vi "send_burleighPairedPulse-v02.vi"(0 "daq_ao":tag="Dev1/ao1", 1 "daq_ai":tag="Dev1/ai0:1", 2 "Jump Polarity":bool, 5 "PairedPulseValuesCluster":T2, 7 "Sample Freq (Hz)":dbl min=0.0 max=40000.0, 12 "Jump Filter Freq (Hz)":dbl=20.0 min=0.0 max=40000.0, 13 "Number of Replicates":i16=1 min=1 max=10, 14 "error in":errorcluster) -> (4 "output cluster":T1, 6 "output waveform":waveform(dbl)[](graph), 8 "protocol response":waveform(dbl)[](graph) caption="jumptestMonitor", 10 "error out":errorcluster)   [LabVIEW 2019]
uses:
  <vilib>/Analysis/3filter.llb/Filter Passband Type.ctl
  <vilib>/Analysis/3filter.llb/Bessel Filter (DBL).vi
  <vilib>/measure/NI_MABase.lvlib
  <vilib>/Analysis/NI_AALBase.lvlib
panel:
  # "doesnt do replicating sweeps, just one go..."
  # "Low"
  # "High"
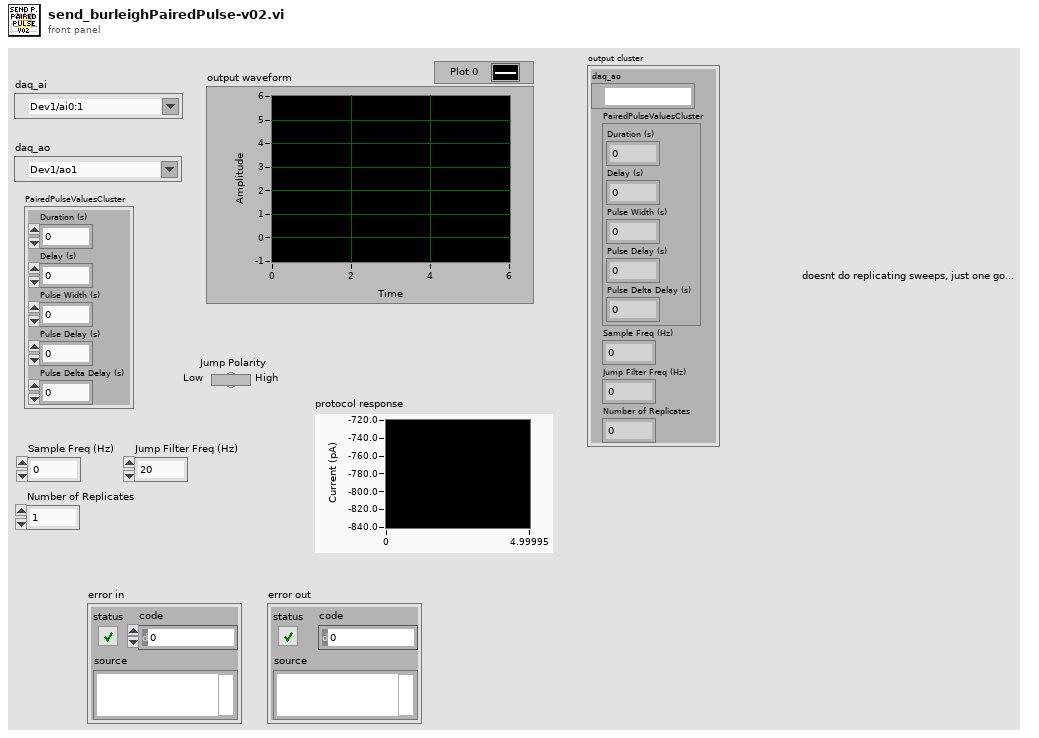
[diagram p1: front panel]
types:
  T1 = cluster{"daq_ao":tag, "PairedPulseValuesCluster":cluster{"Duration (s)":dbl, "Delay (s)":dbl, "Pulse Width (s)":dbl, "Pulse Delay (s)":dbl, "Pulse Delta Delay (s)":dbl}, "Sample Freq (Hz)":dbl, "Jump Filter Freq (Hz)":dbl, "Number of Replicates":i16}
  T2 = cluster{"Duration (s)":dbl, "Delay (s)":dbl, "Pulse Width (s)":dbl, "Pulse Delay (s)":dbl, "Pulse Delta Delay (s)":dbl}
  T3 = typedef "NI_AALBase.lvlib/Filter Passband Type.ctl" = enum32{"Lowpass", "Highpass", "Bandpass", "Bandstop"}
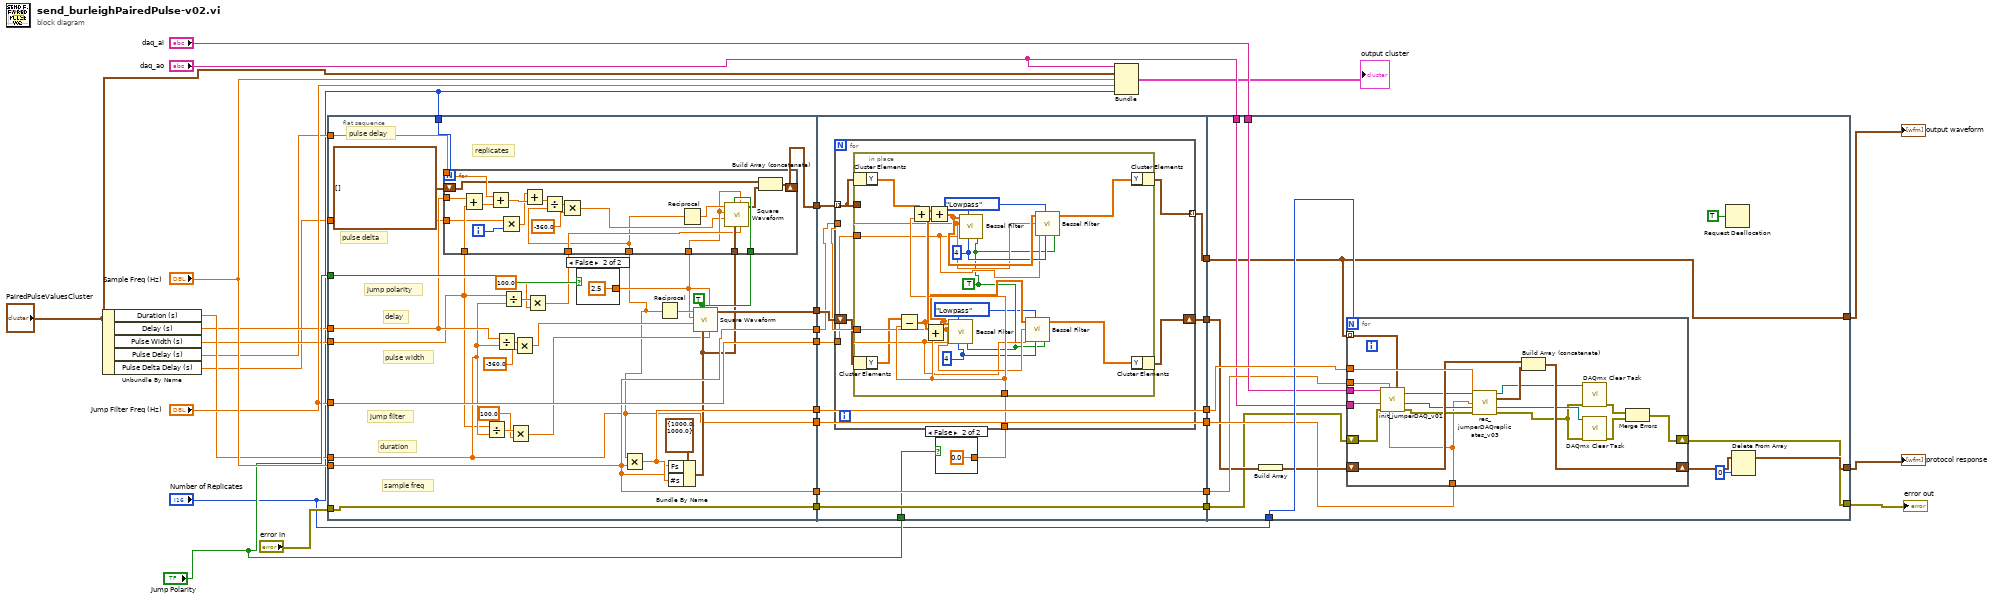
[diagram p0: block diagram]
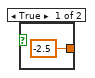
[diagram p2: hidden frame]
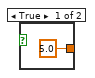
[diagram p3: hidden frame]
diagram:
  n1 = Unbundle By Name("PairedPulseValuesCluster") -> ("Duration (s)"=w10:dbl, "Delay (s)"=w9:dbl, "Pulse Width (s)"=w8:dbl, "Pulse Delay (s)"=w4:dbl, "Pulse Delta Delay (s)"=w2:dbl)
  n2 = flat-sequence {
    tunnel: w10 -> [w34]
    tunnel: "Jump Filter Freq (Hz)" -> [w57]
    tunnel: "Sample Freq (Hz)" -> [w56]
    tunnel: [w58] -> w26
    tunnel: [w56] -> w23
    tunnel: [w57] -> w21
    tunnel: [w56] -> w20
    tunnel: [w55] -> w19
    tunnel: "error in" -> [w54]
    tunnel: [w54] -> w16
    tunnel: "Jump Polarity" -> [w53]
    tunnel: [w34] -> w12
    tunnel: w9 -> [w38]
    tunnel: w8 -> [w33]
    tunnel: [w43] -> w7
    tunnel: w4 -> [w37]
    tunnel: "Number of Replicates" -> [w36]
    tunnel: w2 -> [w35]
    tunnel: w26 -> [w94]
    tunnel: [w94] -> w25
    tunnel: [w92] -> w24
    tunnel: w23 -> [w93]
    tunnel: [w93] -> w22
    tunnel: w21 -> [w86]
    tunnel: w20 -> [w87]
    tunnel: w19 -> [w91]
    tunnel: [w90] -> w17
    tunnel: w16 -> [w90]
    tunnel: "Jump Polarity" -> [w89]
    tunnel: w12 -> [w88]
    tunnel: [w88] -> w11
    tunnel: w7 -> [w84]
    tunnel: [w83] -> w1
    tunnel: [w123] -> w31
    tunnel: w25 -> [w134]
    tunnel: w24 -> [w125]
    tunnel: "daq_ai" -> [w127]
    tunnel: "daq_ao" -> [w124]
    tunnel: w22 -> [w126]
    tunnel: [w130] -> w28
    tunnel: "Number of Replicates" -> [w133]
    tunnel: [w122] -> w15
    tunnel: w17 -> [w121]
    tunnel: w11 -> [w128]
    tunnel: w1 -> [w123]
    frame #0 {
      w47 = TRUE ("reset signal")
      # "replicates"
      # "sample freq"
      # "duration"
      # "jump filter"
      # "pulse width"
      # "delay"
      # "jump polarity"
      # "pulse delta"
      # "pulse delay"
      n3 = Divide(x=w33, y=w34) -> (x/y=w52:dbl)
      n4 = Divide(x=w38, y=w34) -> (x/y=w49:dbl)
      n5 = Divide(x=w33, y=w34) -> (x/y=w45:dbl)
      n6 = Multiply(x=w52, y=100.0) -> (x*y=w41:dbl)
      n7 = Multiply(x=w49, y=-360.0) -> (x*y=w46:dbl)
      n8 = Multiply(x=w45, y=100.0) -> (x*y=w40:dbl)
      n9 = case shown="False" w53 {
        tunnel: [-2.5 ("Amplitude") 2.5 ("Amplitude")] -> w39
        frame True {
        }
        frame False {
        }
      }
      n10 = Multiply(x=w34, y=w56) -> (x*y=w58:dbl)
      n11 = Reciprocal(x=w34) -> (1/x=w48:dbl)
      n12 = Bundle By Name(cluster=cluster{"Fs":dbl, "#s":dbl} {"Fs"=1000.0, "#s"=1000.0} ("sampling info"), "Fs"=w56, "#s"=w58) -> (w42:cluster{"Fs":dbl, "#s":dbl})
      n13 = for {
        N: w36 -> [_]
        tunnel: w47 -> [w80]
        tunnel: w42 -> [w79]
        tunnel: w40 -> [w77]
        tunnel: w39 -> [w76]
        tunnel: w33 -> [w71]
        tunnel: w38 -> [w70]
        tunnel: w37 -> [w69]
        tunnel: w34 -> [w67]
        shift-right: [w65] -> w43
        shift-left: waveform(dbl)[] [] -> [w64]
        tunnel: w35 -> [w60]
        i -> [w62]
        n14 = Add(x=w70, y=w71) -> (x+y=w74:dbl)
        n15 = Add(x=w69, y=w74) -> (x+y=w75:dbl)
        n16 = Multiply(x=w60, y=w62) -> (x*y=w61:dbl)
        n17 = Add(x=w61, y=w75) -> (x+y=w63:dbl)
        n18 = Divide(x=w63, y=w67) -> (x/y=w73:dbl)
        n19 = Multiply(x=w73, y=-360.0) -> (x*y=w72:dbl)
        n20 = Reciprocal(x=w67) -> (1/x=w78:dbl)
        n21 = call <vilib>:"Square Waveform.vi"("duty cycle (%)"=w77, "offset"=w76, "sampling info"=w79, "reset signal"=w80, "phase"=w72, "amplitude"=w76, "frequency"=w78) -> ("signal out"=w66:waveform(dbl))  [unwired: 3 in, 1 out]
        n22 = Build Array (concatenate)(w64, w66) -> (w65:waveform(dbl)[])
      }
      n23 = call <vilib>:"Square Waveform.vi"("duty cycle (%)"=w41, "offset"=w39, "sampling info"=w42, "reset signal"=w47, "phase"=w46, "amplitude"=w39, "frequency"=w48) -> ("signal out"=w55:waveform(dbl))  [unwired: 3 in, 1 out]
    }
    frame #1 {
      n24 = case shown="False" w89 {
        tunnel: [5.0 ("Amplitude") 0.0 ("Amplitude")] -> w85
        frame True {
        }
        frame False {
        }
      }
      n25 = for {
        tunnel: w87 -> [w100]
        tunnel: w86 -> [w99]
        tunnel: w85 -> [w101]
        tunnel: w84 -> [w98] mode=indexing
        shift-right: [w95] -> w92
        shift-left: w91 -> [w96]
        tunnel: [w97] -> w83 mode=indexing
        n26 = in-place {
          in-place-border: w98 -> [_]
          in-place-border: w101 -> [w115]
          in-place-border: w100 -> [w110]
          in-place-border: w99 -> [w109]
          w107 = TRUE ("init/cont (init:F)")
          w112 = 4 ("order")
          w113 = Filter_Passband_Type."Lowpass" ("filter type")
          w108 = 4 ("order")
          w106 = Filter_Passband_Type."Lowpass" ("filter type")
          n27 = in-place-cluster #1(w98) -> ("Y"=w105:dbl[])
          n28 = in-place-cluster #2(w96) -> ("Y"=w103:dbl[])
          n29 = Subtract(x=w103, y=w115) -> (x-y=w116:dbl[])
          n30 = Add(x=w105, y=w115) -> (x+y=w117:dbl[])
          n31 = Add(x=w116, y=w115) -> (x+y=w111:dbl[])
          n32 = Add(x=w117, y=w116) -> (x+y=w114:dbl[])
          n33 = call-poly <vilib>:"Bessel Filter.vi"("init/cont (init:F)"=w107, "order"=w108, "filter type"=w106, "low cutoff freq: fl"=w109, "sampling freq: fs"=w110, "X"=w111) -> ()  [unwired: 2 in, 2 out]
          n34 = call-poly <vilib>:"Bessel Filter.vi"("init/cont (init:F)"=w107, "order"=w112, "filter type"=w113, "low cutoff freq: fl"=w109, "sampling freq: fs"=w110, "X"=w114) -> ()  [unwired: 2 in, 2 out]
          n35 = call-poly <vilib>:"Bessel Filter.vi"("init/cont (init:F)"=w107, "order"=w108, "filter type"=w106, "low cutoff freq: fl"=w109, "sampling freq: fs"=w110, "X"=w111) -> ("Filtered X"=w102:dbl[])  [unwired: 2 in, 1 out]
          n36 = call-poly <vilib>:"Bessel Filter.vi"("init/cont (init:F)"=w107, "order"=w112, "filter type"=w113, "low cutoff freq: fl"=w109, "sampling freq: fs"=w110, "X"=w114) -> ("Filtered X"=w104:dbl[])  [unwired: 2 in, 1 out]
          n37 = in-place-cluster #1("Y"=w104) -> (w97:waveform(dbl))
          n38 = in-place-cluster #2("Y"=w102) -> (w95:waveform(dbl))
        }
      }
    }
    frame #2 {
      n39 = Build Array(w125) -> (w132:waveform(dbl)[])
      n40 = for {
        N: w133 -> [_]
        tunnel: w134 -> [w153]
        shift-right: [w151] -> w131
        shift-left: w132 -> [w150]
        tunnel: w128 -> [w143]
        tunnel: w127 -> [w149]
        tunnel: w126 -> [w148]
        tunnel: w124 -> [w147]
        tunnel: w123 -> [w142] mode=indexing
        shift-right: [w139] -> w122
        shift-left: w121 -> [w138]
        n41 = call "init_jumperDAQ_v01.vi"("protocol waveform"=w142, "Duration (s)"=w143, "Sample Freq (Hz)"=w148, "AO error in"=w138, "AO physical channels"=w147, "AI Physical Channel"=w149) -> ("AO error out"=w146:errorcluster, "AO task out"=w145:refnum<k21>, "AI task out"=w144:refnum<k21>)  [unwired: 1 in, 2 out]
        n42 = call "rec_jumperDAQreplicates_v03.vi"("AI task in"=w144, "number of samples"=w153, "Duration (s)"=w143, "AO task in"=w145, "error in"=w146) -> ("AI task out"=w137:refnum<k21>, "data out (pA or mV)"=w152:waveform(dbl), "AO task out"=w136:refnum<k21>, "error out"=w135:errorcluster)  [unwired: 7 in]
        n43 = Build Array (concatenate)(w150, w152) -> (w151:waveform(dbl)[])
        n44 = call <vilib>:"DAQmx Clear Task.vi"("task in"=w137, "error in"=w135) -> ("error out"=w141:errorcluster)  [unwired: 13 in]
        n45 = call <vilib>:"DAQmx Clear Task.vi"("task in"=w136, "error in"=w135) -> ("error out"=w140:errorcluster)  [unwired: 13 in]
        n46 = Merge Errors(w141, w140) -> (w139:errorcluster)
      }
      n47 = Request Deallocation(TRUE ("flag")) -> ()
      n48 = Delete From Array(array=w131, index=0) -> (array with subset deleted=w130:waveform(dbl)[])  [unwired: 1 in, 1 out]
    }
  }
  n49 = Bundle("daq_ao"="daq_ao", "PairedPulseValuesCluster"="PairedPulseValuesCluster", "Sample Freq (Hz)"="Sample Freq (Hz)", "Jump Filter Freq (Hz)"="Jump Filter Freq (Hz)", "Number of Replicates"="Number of Replicates") -> (→"output cluster":T1)  [unwired: 1 in]
  "protocol response" <- w28
  "output waveform" <- w31
  "error out" <- w15
